vi "Read Act Time.vi"(8 "error in (no error)":errorcluster, 11 "Task Data in":refnum<class "Task Data.lvclass">) -> (0 "error out":errorcluster, 2 "Act Time":sgl, 3 "Task Data out":refnum<class "Task Data.lvclass">)   [LabVIEW 2012, in "Task Data.lvclass"]
uses:
  Task Data.lvclass
  Task Data.lvclass/Task Data.ctl
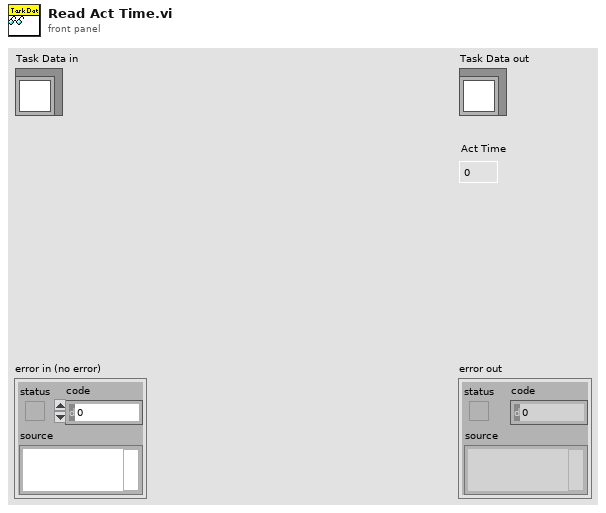
[diagram p1: front panel]
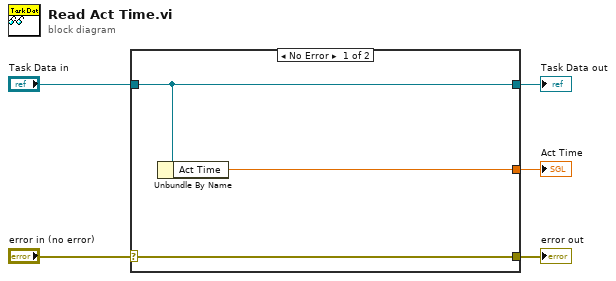
[diagram p0: block diagram]
diagram:
  n1 = case shown="No Error" "error in (no error)" {
    selector: "error in (no error)" -> [w8 w9]
    tunnel: [w8 w9] -> w4
    tunnel: [w7 w10] -> w2
    tunnel: "Task Data in" -> [w7 w10]
    tunnel: [w6 _] -> w1
    frame No Error {
      n2 = Unbundle By Name(w7) -> ("Act Time"=w6:sgl)
    }
    frame Error {
    }
  }
  "error out" <- w4
  "Task Data out" <- w2
  "Act Time" <- w1
